vi "Wait on Stop.vi"(8 "error in (no error)":errorcluster, 11 "MenuButton Event Handler in":refnum<class "MenuButton Event Handler.lvclass">) -> ()   [LabVIEW 2017, in "MenuButtons.lvlib" / "MenuButton Event Handler.lvclass"]
uses:
  MenuButton Event Handler.lvclass
  MenuButton Event Handler.lvclass/MenuButton Event Handler.ctl
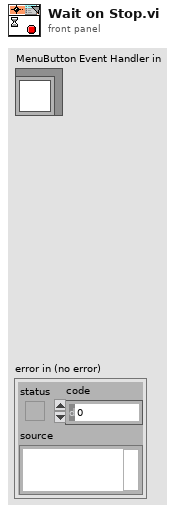
[diagram p1: front panel]
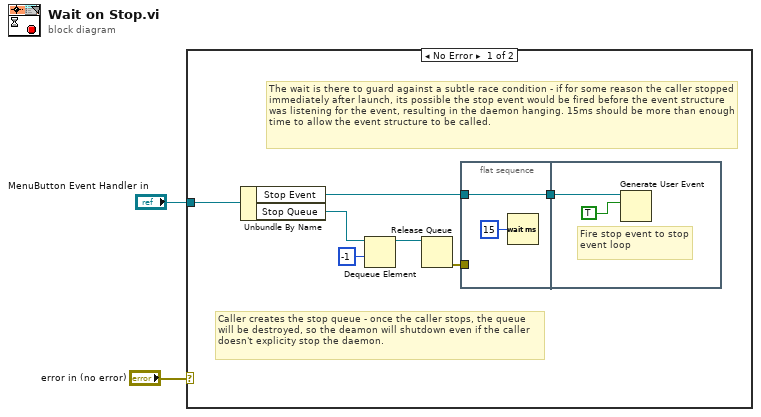
[diagram p0: block diagram]
diagram:
  n1 = case shown="No Error" "error in (no error)" {
    tunnel: "MenuButton Event Handler in" -> [w9 _]
    frame No Error {
      # "The wait is there to guard against a subtle race condition - if for some reason the caller stopped immediately after launch, its possible the stop event would be fired before the event structure was listening for the event, resulting in the daemon hanging. 15ms should be more than enough time to allow the event structure to be called."
      # "Caller creates the stop queue - once the caller stops, the queue will be destroyed, so the deamon will shutdown even if the caller doesn't explicity stop the daemon."
      n2 = Unbundle By Name(w9) -> ("Stop Event"=w7:refnum<user-event>, "Stop Queue"=w8:refnum<queue>)
      n3 = Dequeue Element(queue=w8, timeout in ms (-1)=-1) -> (queue out=w6:refnum<queue>)  [unwired: 1 in, 3 out]
      n4 = Release Queue(queue=w6) -> (error out=w5:errorcluster)  [unwired: 2 in, 2 out]
      n5 = flat-sequence {
        tunnel: w5 -> [_]
        tunnel: w7 -> [w11]
        tunnel: [w11] -> w3
        tunnel: w3 -> [w13]
        frame #0 {
          n6 = Wait (ms)(milliseconds to wait=u32 15) -> ()  [unwired: 1 out]
        }
        frame #1 {
          # "Fire stop event to stop event loop"
          n7 = Generate User Event(user event=w13, event data cluster=TRUE ("event data")) -> ()  [unwired: 2 in, 2 out]
        }
      }
    }
    frame Error {
      # "Do nothing on incoming error"
    }
  }
